vi "Main.vi"() -> ()   [LabVIEW 2013]
doc: "Use this template to build a simple state machine design pattern. Each state executes code and determines which state to transition to."
uses:
  controls/State.ctl
  <vilib>/sound2/lvsound2.llb/Sampling Mode.ctl
  <vilib>/sound2/lvsound2.llb/Sound Data Format.ctl
  <vilib>/Utility/error.llb/DialogType.ctl
  <vilib>/sound2/lvsound2.llb/Sound File Position.ctl
  <vilib>/measure/NI_MAPro.lvlib
  <vilib>/measure/maspectr.llb/FFT Power Spectrum and PSD for 1 Chan.vi
  <vilib>/sound2/lvsound2.llb/Sound Output Write (DBL).vi
  <vilib>/sound2/lvsound2.llb/Sound File Read Open.vi
  <vilib>/sound2/lvsound2.llb/Sound File Info (path).vi
  <vilib>/sound2/lvsound2.llb/Sound File Read (DBL).vi
panel:
  in  "Samples/\nChannel":i32=2000
  out "Spectrum 2":cluster{"f0":dbl, "df":dbl, "magnitude":dbl[]}(graph)
  out "Channel 2":waveform(dbl)(graph)
  out "Spectrum 1":cluster{"f0":dbl, "df":dbl, "magnitude":dbl[]}(graph)
  out "Channel 1":waveform(dbl)(graph)
  in  "?":bool
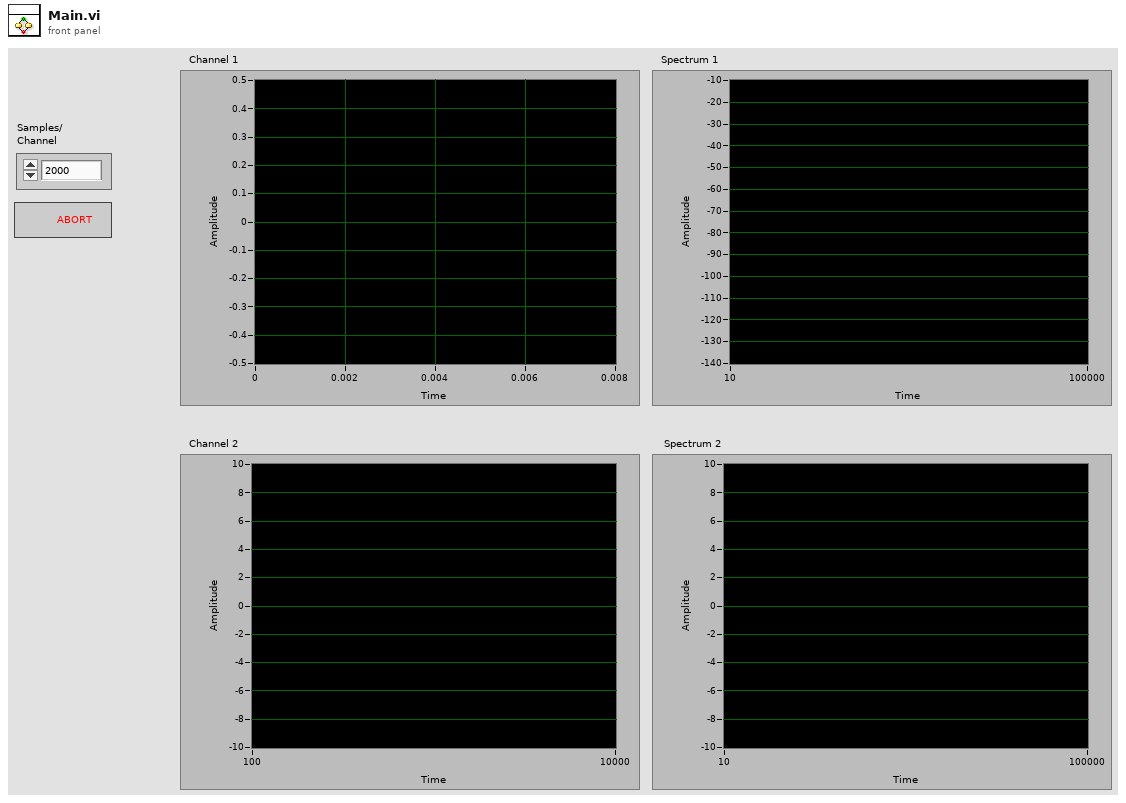
[diagram p1: front panel]
types:
  T1 = typedef "DialogType.ctl" = u16
  T2 = typedef "State.ctl" = enum16{"Setup", "Play", "OpenFile", "Stop"}
  T3 = enum16{"open", "replace", "create", "open or create", "replace or create", "replace or create with confirmation"}
  T4 = typedef "Sound Data Format.ctl" = cluster{"sample rate (S/s)":dbl, "number of channels":i32, "bits per sample":i32}
  T5 = typedef "Sampling Mode.ctl" = i32
  T6 = typedef "Sound Output Task ID.ctl" = u32
  T7 = typedef "Sound File Refnum.ctl" = refnum<file>
  T8 = typedef "Sound File Position.ctl" = u16
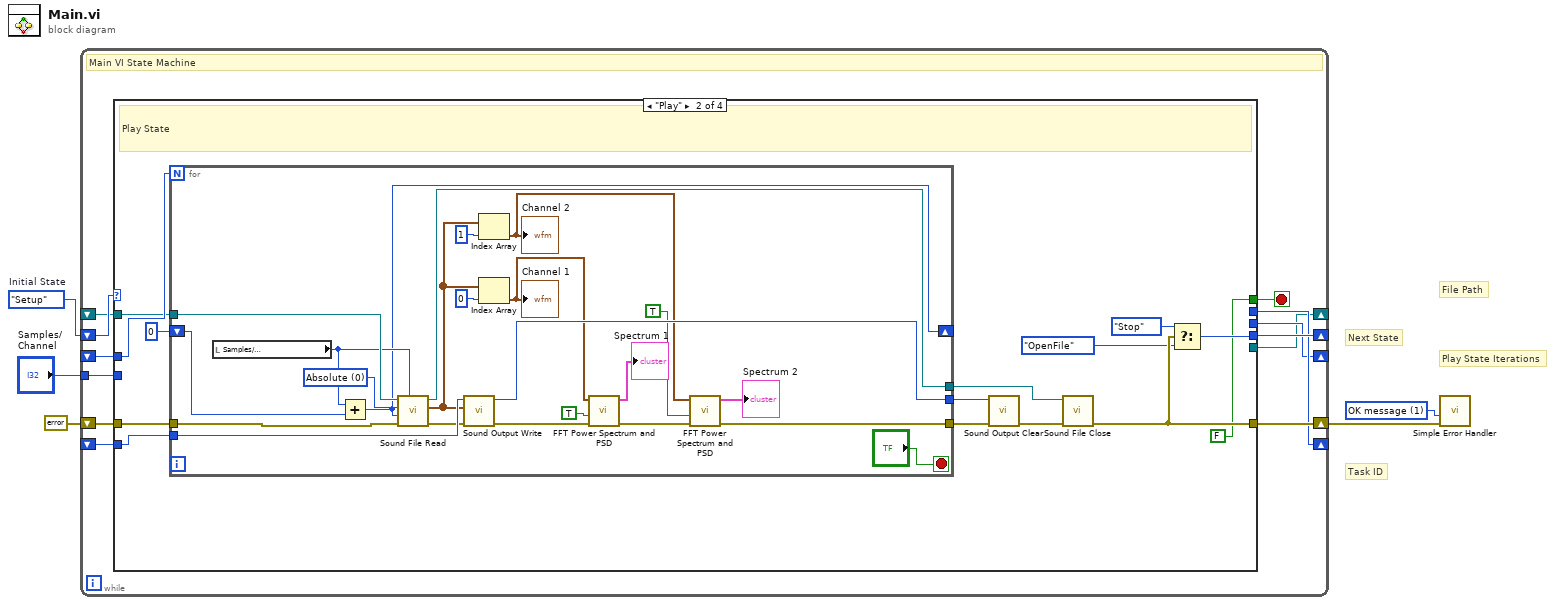
[diagram p0: block diagram]
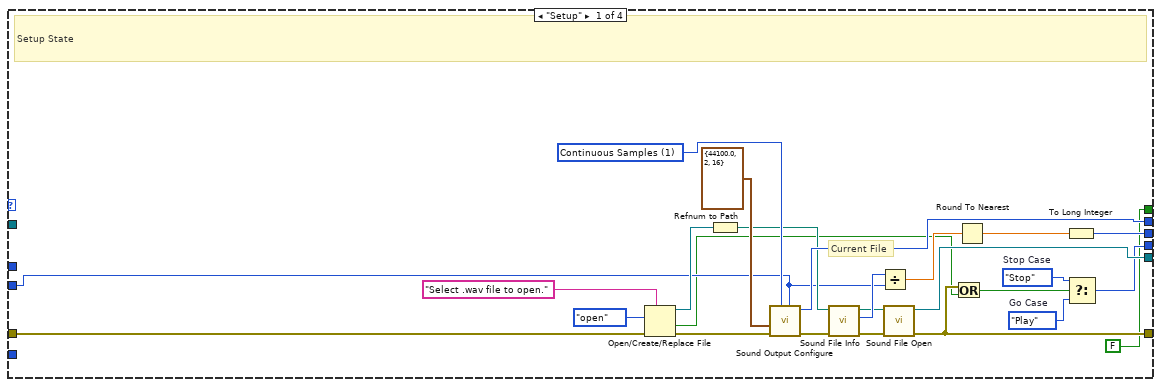
[diagram p2: hidden frame]
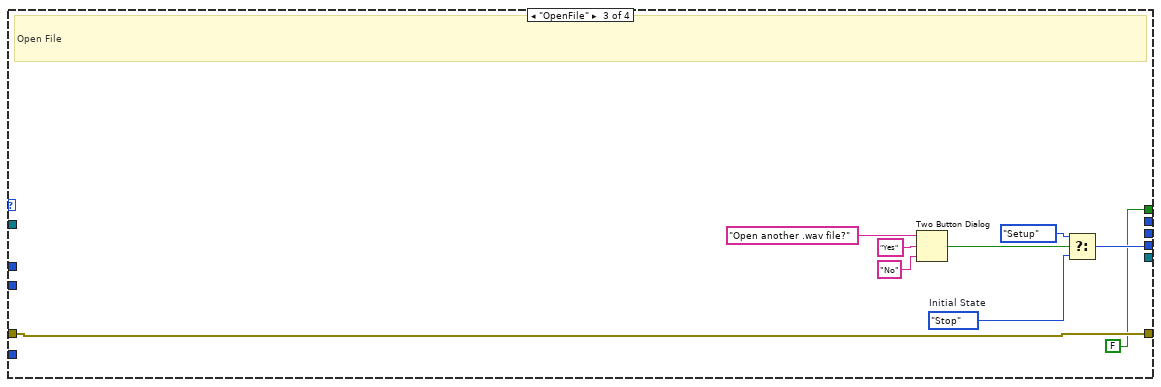
[diagram p3: hidden frame]
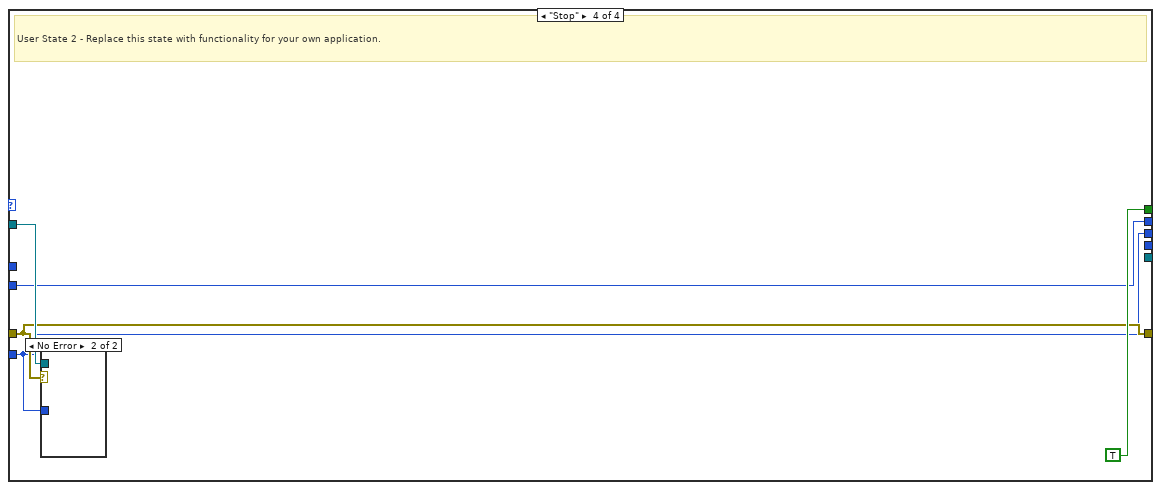
[diagram p4: hidden frame]
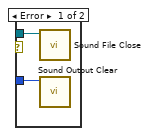
[diagram p5: hidden frame]
diagram:
  w1 = T1 1 items=["no dialog", "OK message", "continue or stop message", "OK message + warnings", "continue/stop + warnings"] ("type of dialog (OK msg:1)")
  w5 = State."Setup"  # Initial State
  # "File Path"
  # "Next State"
  # "Task ID"
  # "Play State Iterations"
  n1 = while {
    shift-right: [w16] -> _
    shift-left: w5 -> [w17]
    shift-right: [w14] -> w2
    shift-left: errorcluster {"status"=FALSE, "code"=0, "source"=""} ("error constant") -> [w15]
    tunnel: "Samples/\nChannel" -> [w13]
    shift-right: [w12] -> _
    shift-left: _ -> [w7]
    shift-right: [w11] -> _
    shift-left: _ -> [w9]
    shift-right: [w10] -> _
    shift-left: _ -> [w8]
    stop <- w6 stop-if-true
    # "Main VI State Machine"
    n2 = case shown="\"Play\"" w17 {
      tunnel: [w22 w56 w81 _] -> w16
      tunnel: w15 -> [w28 w55 w88 w90]
      tunnel: [w21 w54 w88 w90] -> w14
      tunnel: w13 -> [w34 _ _ w91]
      tunnel: [w40 _ _ w91] -> w12
      tunnel: [w31 _ _ w89] -> w11
      tunnel: [w29 _ _ _] -> w10
      tunnel: w9 -> [_ w53 _ _]
      tunnel: w8 -> [_ w52 _ w92]
      tunnel: w7 -> [_ w51 _ w89]
      tunnel: [FALSE FALSE FALSE TRUE] -> w6
      frame "Setup" {
        w23 = State."Play"  # Go Case
        w24 = State."Stop"  # Stop Case
        w42 = T5 1 items=["Finite Samples", "Continuous Samples"] ("sample mode")
        # "Current File"
        # "Setup State"
        n3 = Open/Create/Replace File(error in=w28, prompt="Select .wav file to open.", operation (0:open)=T3."open") -> (refnum out=w37:refnum<file>, cancelled=w20:bool, error out=w27:errorcluster)  [unwired: 3 in]
        n4 = Refnum to Path(1:w37) -> (0:w36:path)
        n5 = call <vilib>:"Sound Output Configure.vi"("number of samples/ch"=w34, "sample mode"=w42, "error in (no error)"=w27, "sound format"=T4 {"sample rate (S/s)"=44100.0, "number of channels"=2, "bits per sample"=16}) -> ("error out"=w26:errorcluster, "task ID"=w40:T6)  [unwired: 6 in]
        n6 = call-poly <vilib>:"Sound File Info.vi"("error in (no error)"=w26, "path"=w36) -> ("error out"=w25:errorcluster, "total number of samples/ch"=w35:u32, "path out"=w30:path)  [unwired: 6 in, 1 out]
        n7 = Divide(x=w35, y=w34) -> (x/y=w33:dbl)
        n8 = call-poly <vilib>:"Sound File Open.vi"("error in (no error)"=w25, "path"=w30) -> ("error out"=w21:errorcluster, "sound file refnum"=w29:T7)  [unwired: 8 in]
        n9 = Or(x=w21, y=w20) -> (x .or. y?=w19:bool)
        n10 = Round To Nearest(number=w33) -> (nearest integer value=w32:dbl)
        n11 = To Long Integer(number=w32) -> (32bit integer=w31:i32)
        n12 = Select(t=w24, s=w19, f=w23) -> (s? t:f=w22:T2)
      }
      frame "Play" {
        # "Play State"
        n13 = for {
          N: w53 -> [_]
          tunnel: w52 -> [w79]
          shift-right: [w75] -> _
          shift-left: 0 -> [w76]
          tunnel: w51 -> [w74]
          tunnel: w55 -> [w73]
          tunnel: [w71] -> w49
          tunnel: [w70] -> w48
          tunnel: [w60] -> w47
          stop <- "?" stop-if-true
          w78 = T8 0 items=["Absolute"=0, "Relative"=2] ("position mode")
          n14 = local read "Samples/\nChannel"() -> (w77:i32)
          n15 = Add(x=w77, y=w76) -> (x+y=w75:i32)
          n16 = call-poly <vilib>:"Sound File Read.vi"("number of samples/ch (-1: all)"=w77, "error in (no error)"=w73, "position offset"=w75, "position mode"=w78, "sound file refnum"=w79) -> ("error out"=w72:errorcluster, "data"=w69:waveform(dbl)[], "sound file refnum out"=w70:T7)  [unwired: 2 in, 2 out]
          n17 = call-poly <vilib>:"Sound Output Write.vi"("error in (no error)"=w72, "data"=w69, "task ID"=w74) -> ("error out"=w62:errorcluster, "task ID out"=w71:T6)  [unwired: 7 in]
          n18 = Index Array(array=w69, index=1) -> (element=w65:waveform(dbl))
          "Channel 2" <- w65
          n19 = Index Array(array=w69, index=0) -> (element=w66:waveform(dbl))
          "Channel 1" <- w66
          n20 = call-poly <vilib>:"FFT Power Spectrum and PSD.vi"("error in (no error)"=w62, "dB On (F)"=TRUE, "time signal"=w66) -> ("error out"=w61:errorcluster, "Power Spectrum / PSD"=→"Spectrum 1":cluster{"f0":dbl, "df":dbl, "magnitude":dbl[]})  [unwired: 5 in, 2 out]
          n21 = call-poly <vilib>:"FFT Power Spectrum and PSD.vi"("error in (no error)"=w61, "dB On (F)"=TRUE, "time signal"=w65) -> ("error out"=w60:errorcluster, "Power Spectrum / PSD"=→"Spectrum 2":cluster{"f0":dbl, "df":dbl, "magnitude":dbl[]})  [unwired: 5 in, 2 out]
        }
        n22 = call <vilib>:"Sound Output Clear.vi"("error in (no error)"=w47, "task ID"=w49) -> ("error out"=w46:errorcluster)  [unwired: 9 in]
        n23 = call <vilib>:"Sound File Close.vi"("error in (no error)"=w46, "sound file refnum"=w48) -> ("error out"=w54:errorcluster)  [unwired: 9 in]
        n24 = Select(t=State."Stop", s=w54, f=State."OpenFile") -> (s? t:f=w56:T2)
      }
      frame "OpenFile" {
        w82 = State."Stop"  # Initial State
        # "Open File"
        n25 = Two Button Dialog(message="Open another .wav file?", 1:"No", 2:"Yes") -> (T button?=w84:bool)
        n26 = Select(t=State."Setup", s=w84, f=w82) -> (s? t:f=w81:T2)
      }
      frame "Stop" {
        # "User State 2 - Replace this state with functionality for your own application."
        n27 = case shown="No Error" w90 {
          tunnel: w92 -> [w94 _]
          tunnel: w89 -> [w95 _]
          frame Error {
            n28 = call <vilib>:"Sound File Close.vi"("sound file refnum"=w94) -> ()  [unwired: 10 in, 1 out]
            n29 = call <vilib>:"Sound Output Clear.vi"("task ID"=w95) -> ()  [unwired: 10 in, 1 out]
          }
          frame No Error {
          }
        }
      }
    }
  }
  n30 = call <vilib>:"Simple Error Handler.vi"("type of dialog (OK msg:1)"=w1, "error in (no error)"=w2) -> ()  [unwired: 3 in, 5 out]
